vi "cluster2json.vi"(8 "error in":errorcluster, 11 "Cluster Ref in":refnum<vi>) -> (0 "error out":errorcluster, 2 "JSON":string, 3 "Cluster Ref out":refnum<vi>)   [LabVIEW 2011, in "JSON.lvlib"]
uses:
  JSON.lvlib
  <vilib>/Utility/GetType.llb/Type Enum.ctl
panel:
  out "value":string
  out "Label.Text":string
  out "Type Enum":T1=enum."String"
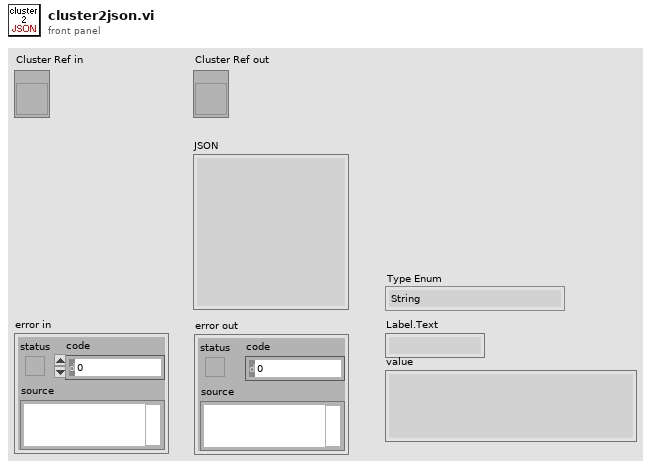
[diagram p1: front panel]
types:
  T1 = typedef "Type Enum.ctl" = enum8{"Void", "I8", "I16", "I32", "I64", "U8", "U16", "U32", "U64", "Single Float", "Double Float", "Extended Float", "Single Complex", "Double Complex", "Extended Complex", "Enum I8 NEVER", "Enum I16 NEVER", "Enum I32 NEVER", "Enum I64 NEVER", "Enum U8", "Enum U16", "Enum U32", "Enum U64", "Single Float With Unit", "Double Float With Unit", "Extended Float With Unit", "Single Complex With Unit", "Double Complex With Unit", "Extended Complex With Unit", "boolU16", "Boolean", "String", "Handle", "Path", "Picture", "C String", "Pascal String", "Tag", "SubString", "Array", "SubArray", "Cluster", "Numeric Cluster", "Variant", "LV Variant", "Measure Data (waveform)", "Refnum", "ExtData", "function", "Typedef", "Poly VI", "bad wire", "LabVIEW Class Instance"}
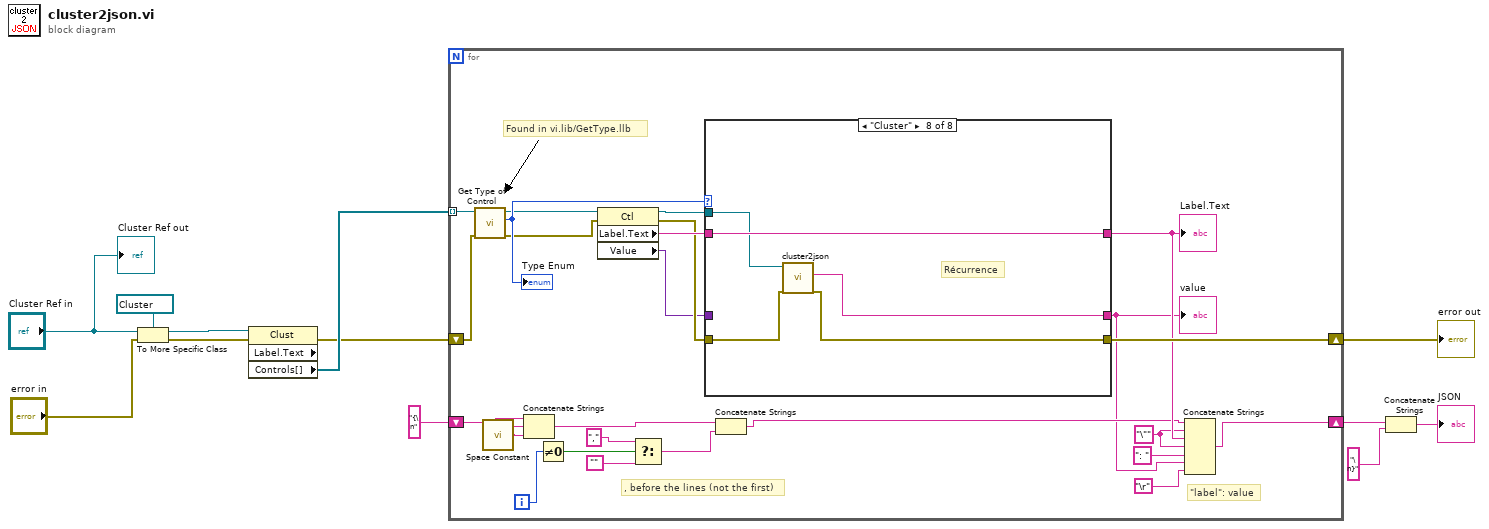
[diagram p0: block diagram]
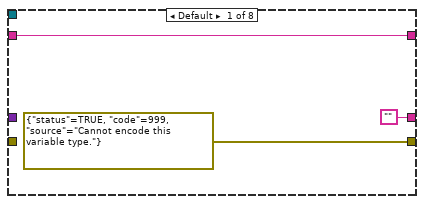
[diagram p2: hidden frame]
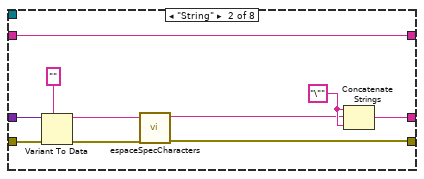
[diagram p3: hidden frame]
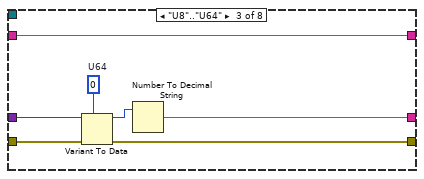
[diagram p4: hidden frame]
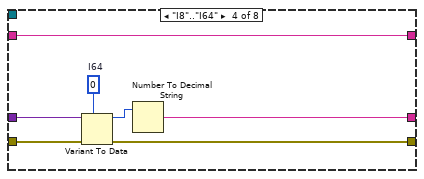
[diagram p5: hidden frame]
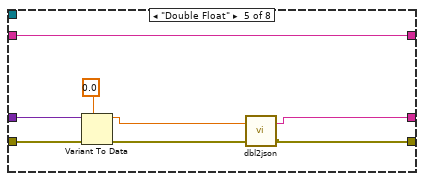
[diagram p6: hidden frame]
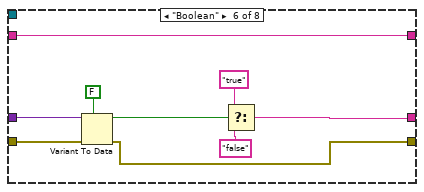
[diagram p7: hidden frame]
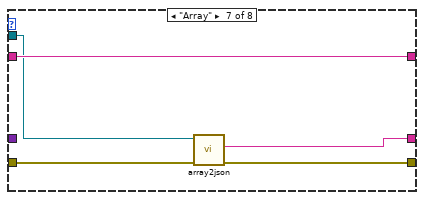
[diagram p8: hidden frame]
diagram:
  n1 = To More Specific Class(target class=refnum<vi> refnum ("reference"), reference="Cluster Ref in", error in="error in") -> (specific class reference=w5:refnum<vi>, error out=w4:errorcluster)
  n2 = property class="Clust" props=["Label", "Text", "Controls[]"](reference=w5, error in=w4) -> (error out=w2:errorcluster, "Controls[]"=w3:refnum<vi>[])  [unwired: 2 out]
  n3 = for {
    shift-right: [w31] -> w10
    shift-left: "{\n" -> [w21]
    tunnel: w3 -> [w15] mode=indexing
    shift-right: [w32] -> w12
    shift-left: w2 -> [w14]
    i -> [w26]
    w28 = "\""
    # ", before the lines (not the first)"
    # "\"label\": value"
    # "Found in vi.lib/GetType.llb"
    n4 = call <vilib>:"Get Type of Control.vi"("error in (no error)"=w14, "Control Ref In"=w15) -> ("error out"=w35:errorcluster, "Type Enum"=w37:T1, "Control Ref Out"=w36:refnum<vi>)  [unwired: 7 in]
    "Type Enum" <- w37
    n5 = call <vilib>:"Space Constant.vi"() -> ("String"=w19:string)
    n6 = Concatenate Strings(w21, w19, w19) -> (w20:string)
    n7 = Not Equal To 0?(x=w26) -> (x != 0?=w27:bool)
    n8 = property class="Ctl"(reference=w36, error in=w35) -> (reference out=w13:refnum<vi>, error out=w33:errorcluster, "Label.Text"=w34:string, "Value"=w18:variant)
    n9 = Select(t=",", s=w27, f="") -> (s? t:f=w25:string)
    n10 = case shown="\"Cluster\"" w37 {
      tunnel: ["" w46 w55 w62 w65 w77 w84 w87] -> w17
      tunnel: [w40 w48 w54 w61 w71 w76 w86 w91] -> w30
      tunnel: w18 -> [_ w49 w53 w60 w69 w74 _ _]
      tunnel: w34 -> [w40 w48 w54 w61 w71 w76 w86 w91]
      tunnel: w33 -> [_ w47 w52 w59 w70 w75 w83 w90]
      tunnel: [errorcluster {"status"=TRUE, "code"=999, "source"="Cannot encode this variable type."} ("error constant") w42 w51 w58 w66 w73 w85 w89] -> w32
      tunnel: w13 -> [_ _ _ _ _ _ w82 w88]
      frame Default {
      }
      frame "String" {
        w45 = "\"" ("search string")
        n11 = Variant To Data(error in=w47, type="", Variant=w49) -> (data=w44:string, error out=w43:errorcluster)
        n12 = call "espaceSpecCharacters.vi"("error in"=w43, "StringIN"=w44) -> ("error out"=w42:errorcluster, "StringOUT"=w41:string)  [unwired: 8 in]
        n13 = Concatenate Strings(w45, w41, w45) -> (w46:string)
      }
      frame "U8".."U64" {
        w57 = u64 0  # U64
        n14 = Variant To Data(error in=w52, type=w57, Variant=w53) -> (data=w56:u64, error out=w51:errorcluster)
        n15 = Number To Decimal String(number=w56) -> (decimal integer string=w55:string)  [unwired: 1 in]
      }
      frame "I8".."I64" {
        w64 = i64 0  # I64
        n16 = Variant To Data(error in=w59, type=w64, Variant=w60) -> (data=w63:i64, error out=w58:errorcluster)
        n17 = Number To Decimal String(number=w63) -> (decimal integer string=w62:string)  [unwired: 1 in]
      }
      frame "Double Float" {
        n18 = Variant To Data(error in=w70, type=0.0, Variant=w69) -> (data=w68:dbl, error out=w67:errorcluster)
        n19 = call "dbl2json.vi"("error in (no error)"=w67, "Numeric"=w68) -> ("error out"=w66:errorcluster, "JSON"=w65:string)
      }
      frame "Boolean" {
        n20 = Variant To Data(error in=w75, type=FALSE, Variant=w74) -> (data=w80:bool, error out=w73:errorcluster)
        n21 = Select(t="true", s=w80, f="false") -> (s? t:f=w77:string)
      }
      frame "Array" {
        n22 = call "array2json.vi"("error in (no error)"=w83, "Array Refnum in"=w82) -> ("error out"=w85:errorcluster, "JSON"=w84:string)  [unwired: 7 in, 1 out]
      }
      frame "Cluster" {
        # "Récurrence"
        n23 = call "cluster2json.vi"("error in"=w90, "Cluster Ref in"=w88) -> ("error out"=w89:errorcluster, "JSON"=w87:string)  [unwired: 7 in, 1 out]
      }
    }
    "Label.Text" <- w30
    "value" <- w17
    n24 = Concatenate Strings(w20, w25) -> (w22:string)
    n25 = Concatenate Strings(w22, w28, w30, w28, ": ", w17, "\r") -> (w31:string)
  }
  "error out" <- w12
  n26 = Concatenate Strings(w10, "\n}") -> (→"JSON":string)
  "Cluster Ref out" <- "Cluster Ref in"
